vi "Quiz1.vi"() -> ()   [LabVIEW 2020]
panel:
  in  "Nk 12":string
  in  "Nk 11":string
  in  "Nk 10":string
  in  "Nk 9":string
  in  "Nk 8":string
  in  "Nk 7":string
  in  "Nk 6":string
  in  "Nk 5":string
  in  "Nk 4":string
  in  "Nk 3":string
  in  "Nk 2":string
  in  "Nk":string
  in  "Sys 12":string
  in  "Sys 11":string
  in  "Sys 10":string
  in  "Sys 9":string
  in  "Sys 8":string
  in  "Sys 7":string
  in  "Sys 6":string
  in  "Sys 5":string
  in  "Sys 4":string
  in  "Sys 3":string
  in  "Sys 2":string
  in  "Tab Control":T1(tab)
  in  "Acceder":bool
  in  "Contraseña":string
  in  "Usuario":string
  in  "OK Button 10":bool
  in  "Sys":string
  in  "Log time(s)":string
  in  "RTU Device ID":string
  in  "Report period(s)":string
  in  "Connection timeout(s)":string
  in  "TCP Port":string
  in  "Low Pass Silter Pole":string
  in  "Zero Offser(AC channels)":string
  in  "Calibration Again(AC channels)":string
  in  "Sampling(s)":string
  in  "RTU Parity":string(combo)
  in  "RTU BaudRate":string(combo)
  in  "Validated address":string
  in  "IP or hostname":string
  in  "Channel(0)":bool
  in  "Channel(1)":bool
  in  "Channel(2)":bool
  in  "OK Button 5":bool
  in  "OK Button 6":bool
  in  "Default Modem Device":i8
  in  "APN":string
  in  "LAN Priority":string(combo)
  in  "Ethernet routher":string
  in  "Ethernet IP Address":string
  in  "WLAN Priority":string(combo)
  in  "Wifi router":string
  in  "Wifi IP Address":string
  in  "Wifi Password":string
  in  "SSID":string
  in  "OK Button 11":bool
  in  "OK Button 8":bool
  in  "OK Button 7":bool
  in  "?":string
  in  "OK Button 9":bool
  in  "String":string
  # "Remote report"
  # "AC channels adjustments"
  # "DC Channels:"
  # "Modbus RTU(Rs-485)"
  # "Wifi Connection"
  # "Ethernet Connection"
  # "Cellular Connection(High priority)"
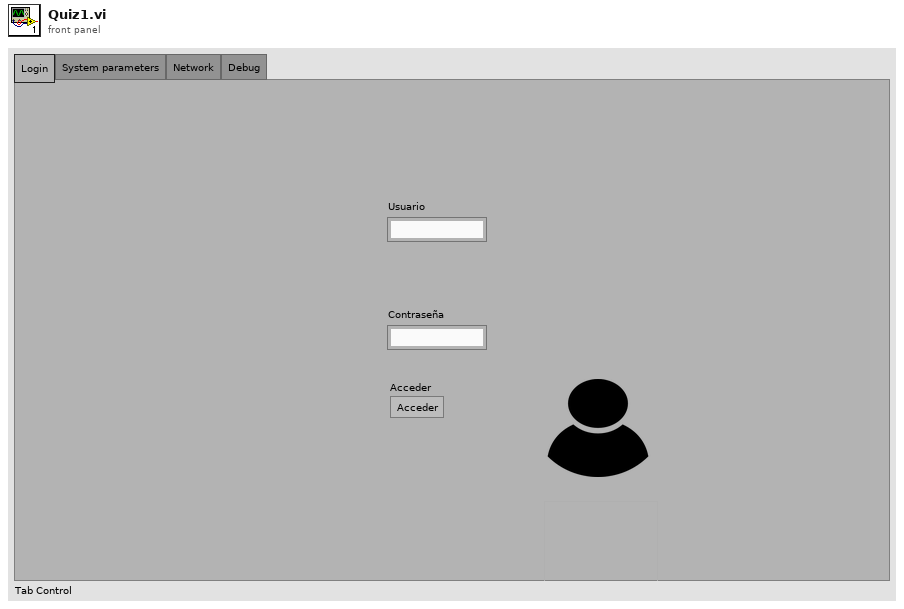
[diagram p1: front panel]
types:
  T1 = enum32{"Login", "System parameters", "Network", "Debug"}
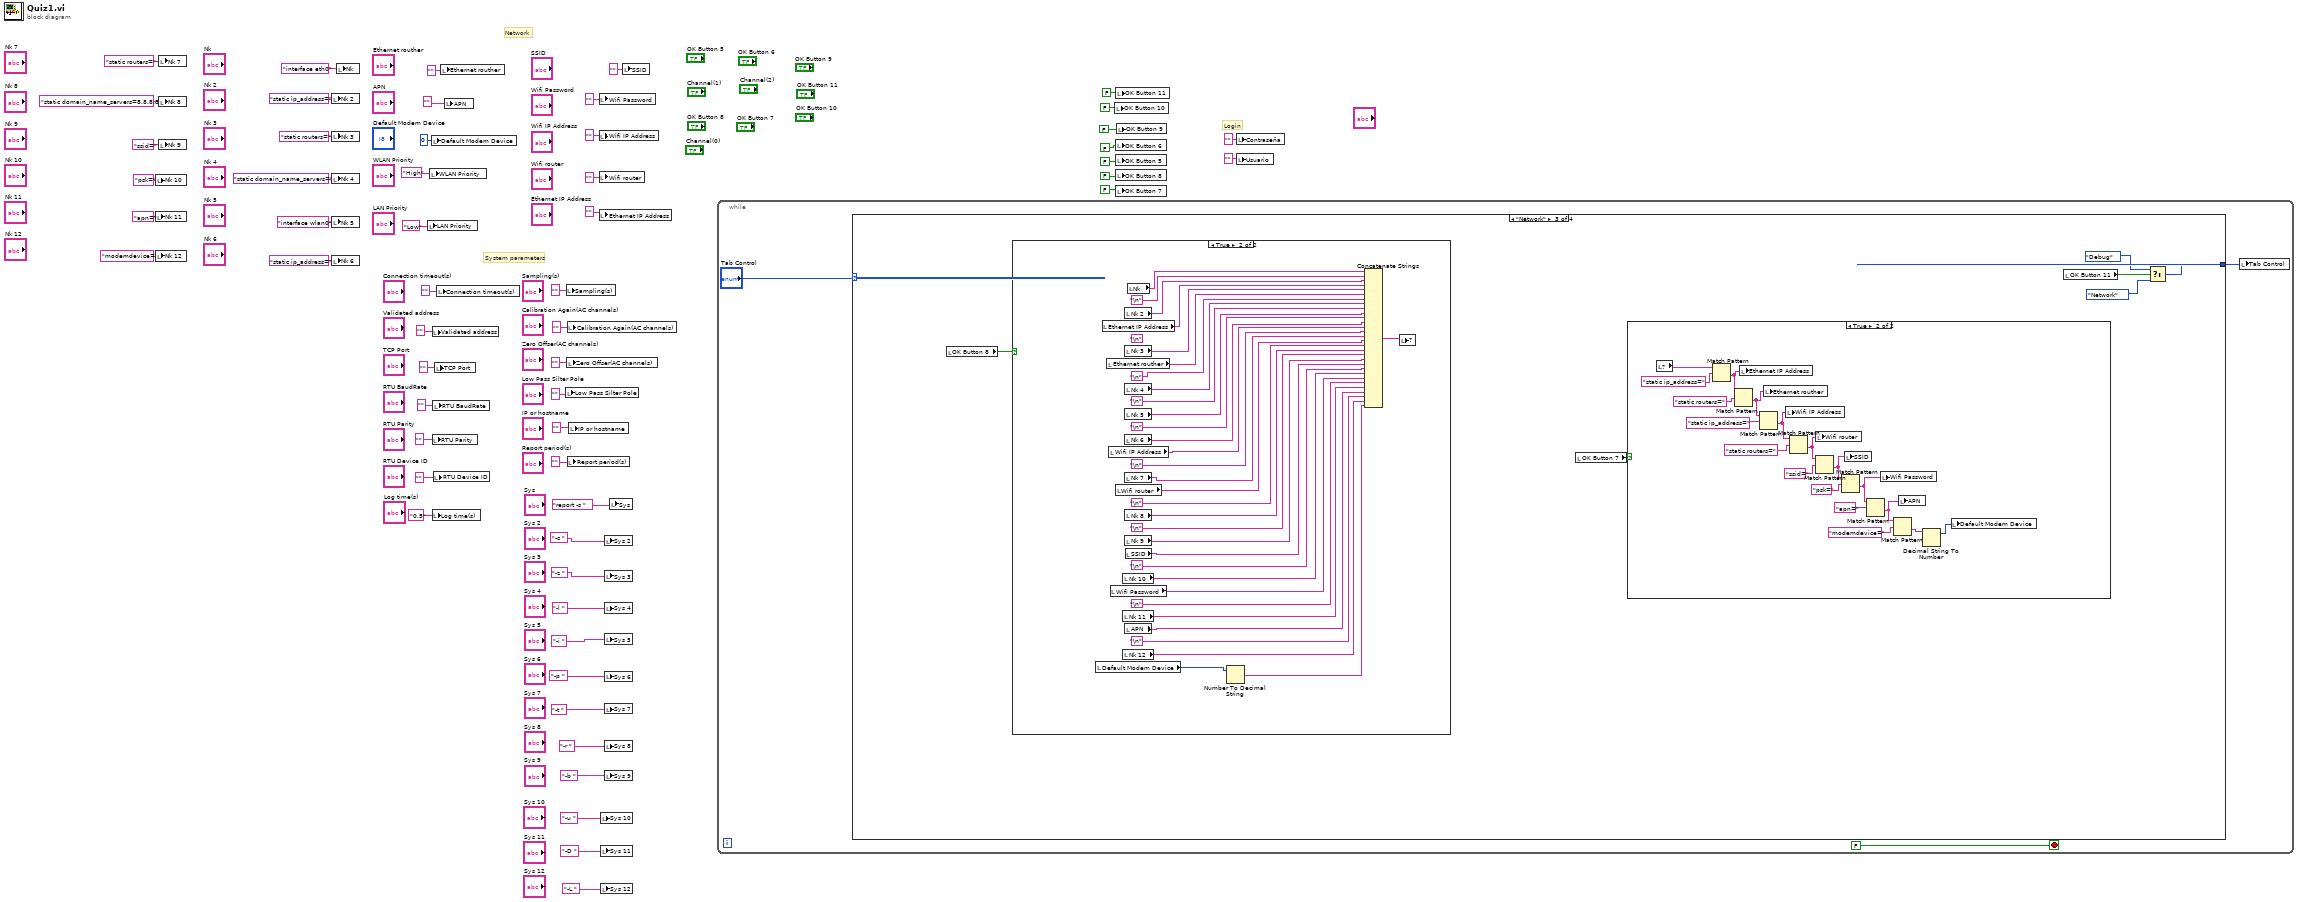
[diagram p0: block diagram]
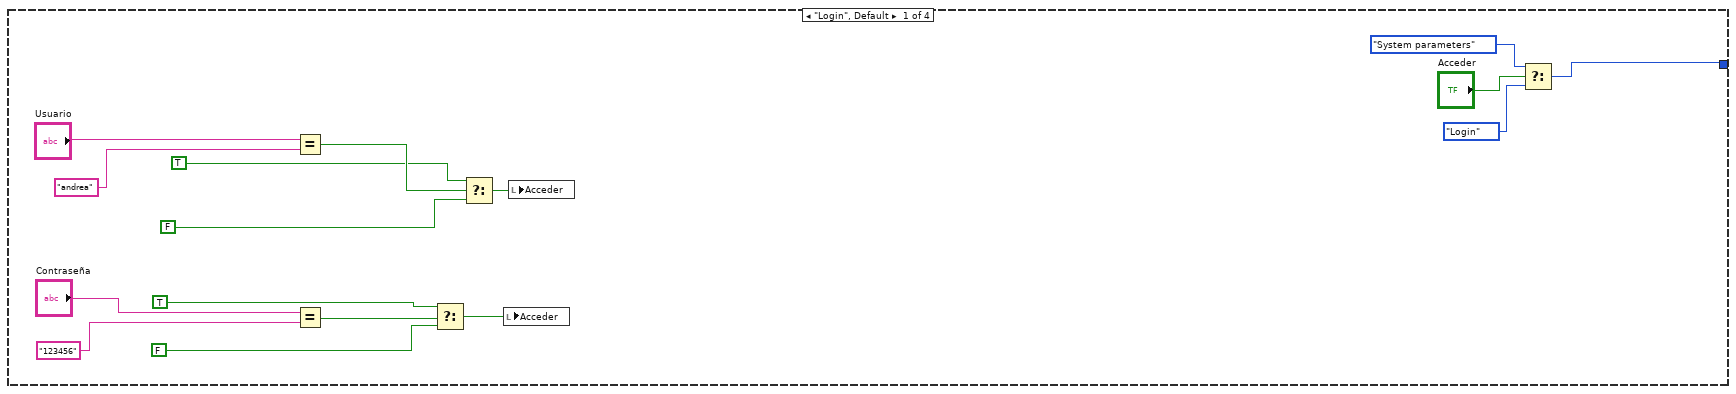
[diagram p2: hidden frame]
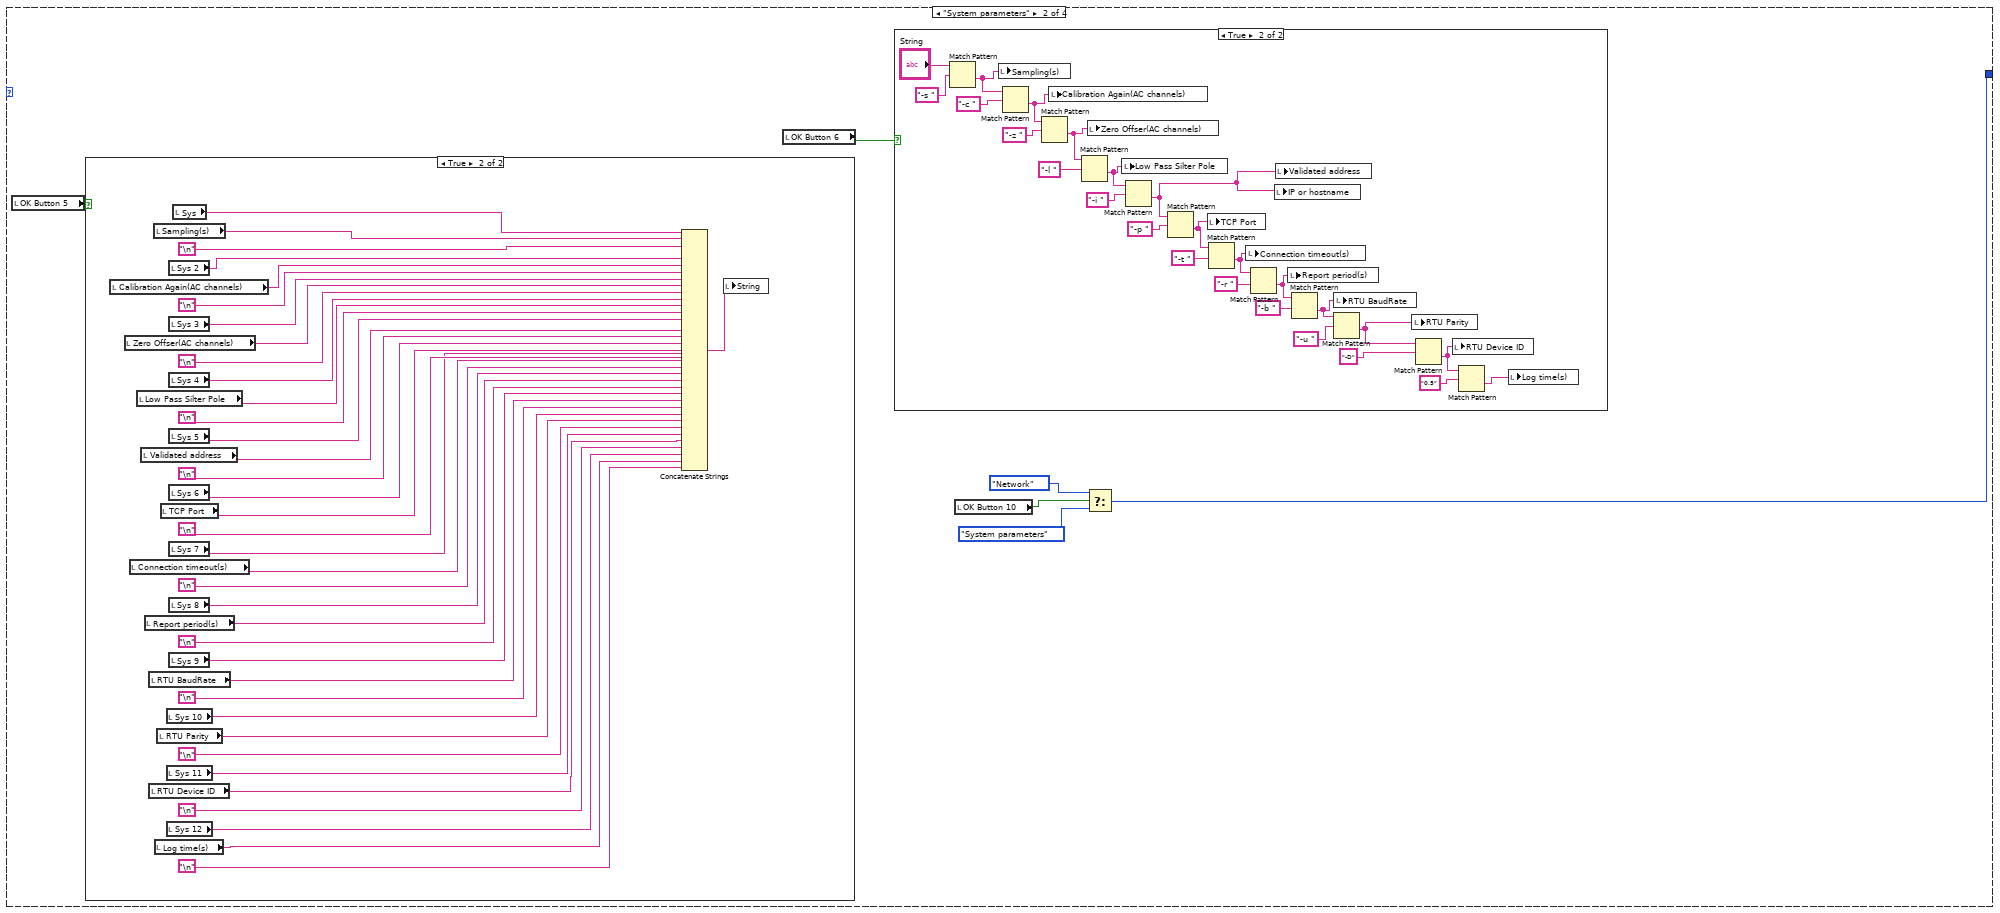
[diagram p3: hidden frame]
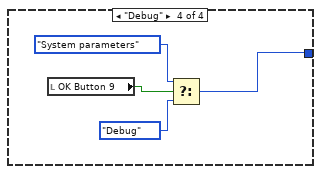
[diagram p8: hidden frame]
diagram:
  # "System parameters"
  # "Network"
  # "Login"
  n1 = local write "Nk 10"("psk=" ("Nk 10")) -> ()
  n2 = local write "Nk 11"("apn=" ("Nk 11")) -> ()
  n3 = local write "Nk 12"("modemdevice=" ("Nk 12")) -> ()
  n4 = local write "Nk 7"("static routers=" ("Nk 7")) -> ()
  n5 = local write "Nk 8"("static domain_name_servers=8.8.8.8" ("Nk 8")) -> ()
  n6 = local write "Nk 9"("ssid=" ("Nk 9")) -> ()
  n7 = local write "Nk 2"("static ip_address=" ("Nk 2")) -> ()
  n8 = local write "Nk 3"("static routers=" ("Nk 3")) -> ()
  n9 = local write "Nk 4"("static domain_name_servers=" ("Nk 4")) -> ()
  n10 = local write "Nk 5"("interface wlan0" ("Nk 5")) -> ()
  n11 = local write "Nk 6"("static ip_address=" ("Nk 6")) -> ()
  n12 = local write "Nk"("interface eth0" ("Nk")) -> ()
  n13 = local write "LAN Priority"("Low" ("Wifi Password")) -> ()
  n14 = local write "WLAN Priority"("High" ("Wifi Password")) -> ()
  n15 = local write "Default Modem Device"(i8 0 ("Default Modem Device")) -> ()
  n16 = local write "Validated address"("" ("Connection timeout(s)")) -> ()
  n17 = local write "RTU Parity"("" ("Connection timeout(s)")) -> ()
  n18 = local write "Log time(s)"("0.5" ("Connection timeout(s)")) -> ()
  n19 = local write "RTU BaudRate"("" ("Connection timeout(s)")) -> ()
  n20 = local write "RTU Device ID"("" ("Connection timeout(s)")) -> ()
  n21 = local write "TCP Port"("" ("Connection timeout(s)")) -> ()
  n22 = local write "Connection timeout(s)"("" ("Connection timeout(s)")) -> ()
  n23 = local write "Ethernet routher"("" ("Wifi Password")) -> ()
  n24 = local write "APN"("" ("Wifi Password")) -> ()
  n25 = local write "Low Pass Silter Pole"("" ("Connection timeout(s)")) -> ()
  n26 = local write "Sampling(s)"("" ("Connection timeout(s)")) -> ()
  n27 = local write "Zero Offser(AC channels)"("" ("Connection timeout(s)")) -> ()
  n28 = local write "Calibration Again(AC channels)"("" ("Connection timeout(s)")) -> ()
  n29 = local write "Report period(s)"("" ("Connection timeout(s)")) -> ()
  n30 = local write "IP or hostname"("" ("Connection timeout(s)")) -> ()
  n31 = local write "Wifi Password"("" ("Wifi Password")) -> ()
  n32 = local write "Wifi IP Address"("" ("Wifi Password")) -> ()
  n33 = local write "Wifi router"("" ("Wifi Password")) -> ()
  n34 = local write "Ethernet IP Address"("" ("Wifi Password")) -> ()
  n35 = local write "Sys 10"("-u " ("Sys 10")) -> ()
  n36 = local write "Sys 11"("-D " ("Sys 11")) -> ()
  n37 = local write "Sys 12"("-L " ("Sys 12")) -> ()
  n38 = local write "Sys 2"("-c " ("Connection timeout(s)")) -> ()
  n39 = local write "Sys 3"("-z " ("Connection timeout(s)")) -> ()
  n40 = local write "Sys 4"("-l " ("Connection timeout(s)")) -> ()
  n41 = local write "Sys 5"("-i " ("Connection timeout(s)")) -> ()
  n42 = local write "Sys 6"("-p " ("Connection timeout(s)")) -> ()
  n43 = local write "Sys 7"("-t " ("Connection timeout(s)")) -> ()
  n44 = local write "Sys 8"("-r " ("Sys 8")) -> ()
  n45 = local write "Sys 9"("-b " ("Sys 9")) -> ()
  n46 = local write "Sys"("report -s " ("Connection timeout(s)")) -> ()
  n47 = local write "SSID"("" ("SSID")) -> ()
  n48 = while {
    stop <- FALSE stop-if-true
    n49 = case shown="\"Network\"" "Tab Control" {
      tunnel: [w60 w81 w147 w200] -> w57
      frame "Login", Default {
        n50 = Equal?(x="Usuario", y="andrea") -> (x = y?=w71:bool)
        n51 = Equal?(x="Contraseña", y="123456") -> (x = y?=w70:bool)
        n52 = Select(t=TRUE, s=w70, f=FALSE) -> (s? t:f=w64:bool)
        n53 = Select(t=TRUE, s=w71, f=FALSE) -> (s? t:f=w65:bool)
        n54 = local write "Acceder"(w64) -> ()
        n55 = local write "Acceder"(w65) -> ()
        n56 = Select(t=T1."System parameters" ("Tab Control"), s="Acceder", f=T1."Login" ("Tab Control")) -> (s? t:f=w60:T1)
      }
      frame "System parameters" {
        n57 = local read "OK Button 5"() -> (w77:bool)
        n58 = case shown="True" w77 {
          frame False {
          }
          frame True {
            n59 = local read "Calibration Again(AC channels)"() -> (w113:string)
            n60 = local read "Zero Offser(AC channels)"() -> (w110:string)
            n61 = local read "Connection timeout(s)"() -> (w98:string)
            n62 = local read "Low Pass Silter Pole"() -> (w107:string)
            n63 = local read "Validated address"() -> (w104:string)
            n64 = local read "Report period(s)"() -> (w95:string)
            n65 = local read "RTU BaudRate"() -> (w92:string)
            n66 = local read "RTU Device ID"() -> (w86:string)
            n67 = local read "Sampling(s)"() -> (w116:string)
            n68 = local read "Log time(s)"() -> (w83:string)
            n69 = local read "RTU Parity"() -> (w89:string)
            n70 = local read "TCP Port"() -> (w101:string)
            n71 = local read "Sys 10"() -> (w90:string)
            n72 = local read "Sys 11"() -> (w87:string)
            n73 = local read "Sys 12"() -> (w84:string)
            n74 = local read "Sys 2"() -> (w114:string)
            n75 = local read "Sys 3"() -> (w111:string)
            n76 = local read "Sys 4"() -> (w108:string)
            n77 = local read "Sys 5"() -> (w105:string)
            n78 = local read "Sys 6"() -> (w102:string)
            n79 = local read "Sys 7"() -> (w99:string)
            n80 = local read "Sys 8"() -> (w96:string)
            n81 = local read "Sys 9"() -> (w93:string)
            n82 = local read "Sys"() -> (w117:string)
            n83 = Concatenate Strings(w117, w116, "\n", w114, w113, "\n", w111, w110, "\n", w108, w107, "\n", w105, w104, "\n", w102, w101, "\n", w99, w98, "\n", w96, w95, "\n", w93, w92, "\n", w90, w89, "\n", w87, w86, "\n", w84, w83, "\n") -> (w118:string)
            n84 = local write "String"(w118) -> ()
          }
        }
        n85 = local read "OK Button 6"() -> (w78:bool)
        n86 = case shown="True" w78 {
          frame False {
          }
          frame True {
            n87 = Match Pattern(string="String", regular expression="-s " ("IP or hostname")) -> (after substring=w130:string)  [unwired: 1 in, 3 out]
            n88 = local write "Sampling(s)"(w130) -> ()
            n89 = Match Pattern(string=w130, regular expression="-c ") -> (after substring=w129:string)  [unwired: 1 in, 3 out]
            n90 = Match Pattern(string=w129, regular expression="-z ") -> (after substring=w128:string)  [unwired: 1 in, 3 out]
            n91 = local write "Calibration Again(AC channels)"(w129) -> ()
            n92 = Match Pattern(string=w128, regular expression="-l ") -> (after substring=w127:string)  [unwired: 1 in, 3 out]
            n93 = local write "Zero Offser(AC channels)"(w128) -> ()
            n94 = local write "Low Pass Silter Pole"(w127) -> ()
            n95 = Match Pattern(string=w127, regular expression="-i ") -> (after substring=w126:string)  [unwired: 1 in, 3 out]
            n96 = Match Pattern(string=w126, regular expression="-p ") -> (after substring=w125:string)  [unwired: 1 in, 3 out]
            n97 = local write "TCP Port"(w125) -> ()
            n98 = Match Pattern(string=w125, regular expression="-t ") -> (after substring=w124:string)  [unwired: 1 in, 3 out]
            n99 = local write "Connection timeout(s)"(w124) -> ()
            n100 = Match Pattern(string=w124, regular expression="-r ") -> (after substring=w123:string)  [unwired: 1 in, 3 out]
            n101 = local write "IP or hostname"(w126) -> ()
            n102 = local write "Validated address"(w126) -> ()
            n103 = local write "Report period(s)"(w123) -> ()
            n104 = Match Pattern(string=w123, regular expression="-b ") -> (after substring=w122:string)  [unwired: 1 in, 3 out]
            n105 = Match Pattern(string=w122, regular expression="-u ") -> (after substring=w121:string)  [unwired: 1 in, 3 out]
            n106 = local write "RTU BaudRate"(w122) -> ()
            n107 = local write "RTU Parity"(w121) -> ()
            n108 = Match Pattern(string=w121, regular expression="-D") -> (after substring=w120:string)  [unwired: 1 in, 3 out]
            n109 = local write "RTU Device ID"(w120) -> ()
            n110 = Match Pattern(string=w120, regular expression="0.5") -> (after substring=w119:string)  [unwired: 1 in, 3 out]
            n111 = local write "Log time(s)"(w119) -> ()
          }
        }
        n112 = local read "OK Button 10"() -> (w76:bool)
        n113 = Select(t=T1."Network" ("Tab Control"), s=w76, f=T1."System parameters" ("Tab Control")) -> (s? t:f=w81:T1)
      }
      frame "Network" {
        n114 = local read "OK Button 8"() -> (w145:bool)
        n115 = case shown="True" w145 {
          frame False {
          }
          frame True {
            (unwired) "\n"
            n116 = local read "Default Modem Device"() -> (w170:i8)
            n117 = local read "Ethernet IP Address"() -> (w196:string)
            n118 = local read "Ethernet routher"() -> (w194:string)
            n119 = local read "Wifi IP Address"() -> (w187:string)
            n120 = local read "Wifi Password"() -> (w176:string)
            n121 = local read "Wifi router"() -> (w184:string)
            n122 = local read "Nk 10"() -> (w177:string)
            n123 = local read "Nk 11"() -> (w174:string)
            n124 = local read "Nk 12"() -> (w171:string)
            n125 = local read "Nk 2"() -> (w197:string)
            n126 = local read "Nk 3"() -> (w195:string)
            n127 = local read "Nk 4"() -> (w192:string)
            n128 = local read "Nk 5"() -> (w190:string)
            n129 = local read "Nk 6"() -> (w188:string)
            n130 = local read "Nk 7"() -> (w185:string)
            n131 = local read "Nk 8"() -> (w182:string)
            n132 = local read "Nk 9"() -> (w180:string)
            n133 = local read "APN"() -> (w173:string)
            n134 = local read "SSID"() -> (w179:string)
            n135 = local read "Nk"() -> (w199:string)
            n136 = Number To Decimal String(number=w170) -> (decimal integer string=w169:string)  [unwired: 1 in]
            n137 = Concatenate Strings(w199, "\n", w197, w196, w195, w194, "\n", w192, "\n", w190, "\n", w188, w187, "\n", w185, w184, "\n", w182, "\n", w180, w179, "\n", w177, w176, "\n", w174, w173, "\n", w171, w169) -> (w168:string)
            n138 = local write item#62(w168) -> ()
          }
        }
        n139 = local read "OK Button 7"() -> (w144:bool)
        n140 = case shown="True" w144 {
          frame False {
          }
          frame True {
            n141 = local read item#62() -> (w150:string)
            n142 = Match Pattern(string=w150, regular expression="static ip_address=" ("IP or hostname")) -> (after substring=w166:string)  [unwired: 1 in, 3 out]
            n143 = Match Pattern(string=w166, regular expression="static routers=" ("IP or hostname")) -> (after substring=w160:string)  [unwired: 1 in, 3 out]
            n144 = local write "Ethernet IP Address"(w166) -> ()
            n145 = Match Pattern(string=w160, regular expression="static ip_address=" ("IP or hostname")) -> (after substring=w159:string)  [unwired: 1 in, 3 out]
            n146 = local write "Ethernet routher"(w160) -> ()
            n147 = local write "Wifi IP Address"(w159) -> ()
            n148 = Match Pattern(string=w159, regular expression="static routers=" ("IP or hostname")) -> (after substring=w158:string)  [unwired: 1 in, 3 out]
            n149 = local write "Wifi router"(w158) -> ()
            n150 = Match Pattern(string=w158, regular expression="ssid=" ("IP or hostname")) -> (after substring=w157:string)  [unwired: 1 in, 3 out]
            n151 = Match Pattern(string=w157, regular expression="psk=" ("IP or hostname")) -> (after substring=w156:string)  [unwired: 1 in, 3 out]
            n152 = local write "SSID"(w157) -> ()
            n153 = Match Pattern(string=w156, regular expression="apn=" ("IP or hostname")) -> (after substring=w153:string)  [unwired: 1 in, 3 out]
            n154 = local write "Wifi Password"(w156) -> ()
            n155 = Match Pattern(string=w153, regular expression="modemdevice=" ("IP or hostname")) -> (after substring=w152:string)  [unwired: 1 in, 3 out]
            n156 = local write "APN"(w153) -> ()
            n157 = Decimal String To Number(string=w152) -> (offset past number=w151:i32)  [unwired: 2 in, 1 out]
            n158 = local write "Default Modem Device"(w151) -> ()
          }
        }
        n159 = local read "OK Button 11"() -> (w146:bool)
        n160 = Select(t=T1."Debug" ("Tab Control"), s=w146, f=T1."Network" ("Tab Control")) -> (s? t:f=w147:T1)
      }
      frame "Debug" {
        n161 = local read "OK Button 9"() -> (w203:bool)
        n162 = Select(t=T1."System parameters" ("Tab Control"), s=w203, f=T1."Debug" ("Tab Control")) -> (s? t:f=w200:T1)
      }
    }
    n163 = local write "Tab Control"(w57) -> ()
  }
  n164 = local write "OK Button 10"(FALSE ("OK Button 10")) -> ()
  n165 = local write "OK Button 11"(FALSE ("OK Button 11")) -> ()
  n166 = local write "OK Button 6"(FALSE ("OK Button 8")) -> ()
  n167 = local write "OK Button 5"(FALSE ("OK Button 8")) -> ()
  n168 = local write "OK Button 8"(FALSE ("OK Button 8")) -> ()
  n169 = local write "OK Button 7"(FALSE ("OK Button 8")) -> ()
  n170 = local write "OK Button 9"(FALSE ("OK Button 8")) -> ()
  n171 = local write "Contraseña"("" ("Contraseña")) -> ()
  n172 = local write "Usuario"("" ("Usuario")) -> ()
